vi "safe state action.vi"(8 "error in":errorcluster, 11 "Engine Data Out in":T1={"timed loop timer source"={"Processor"=0, "Priority"=0, "timing source dt"=0, "timer source"=refnum}, "control loop data"={"engine tag bus"={"Double"=[], "Single"=[], "I64"=[], "I32"=[], "I16"=[], "I8"=[], "U64"=[], "U32"=[], "U16"=[], "U8"=[], "Boolean"=[], "String"=[], "Array of Double"=[], "Array of Single"=[], "Array of I64"=[], "Array of I32"=[], "Array of I16"=[], "Array of I8"=[], "Array of U64"=[], "Array of U32"=[], "Array of U16"=[], "Array of U8"=[], "Array of Boolean"=[], "Array of String"=[]}, "engine schedule"={"module run flags"=[], "decimation schedule"={"decimations"=[], "offsets"=[]}}, "module information"=[]}, "status reporting"={"late? index (bool)"=-1, "late count index (U32)"=-1, "dt (ns) index (U64)"=-1}} {"control loop data"."module information"."GUID"."Lo" format="%.0x"; "control loop data"."module information"."GUID"."Hi" format="%.0x"}) -> (0 "error out":errorcluster, 3 "Engine Data Out out":T1={"timed loop timer source"={"Processor"=0, "Priority"=0, "timing source dt"=0, "timer source"=refnum}, "control loop data"={"engine tag bus"={"Double"=[], "Single"=[], "I64"=[], "I32"=[], "I16"=[], "I8"=[], "U64"=[], "U32"=[], "U16"=[], "U8"=[], "Boolean"=[], "String"=[], "Array of Double"=[], "Array of Single"=[], "Array of I64"=[], "Array of I32"=[], "Array of I16"=[], "Array of I8"=[], "Array of U64"=[], "Array of U32"=[], "Array of U16"=[], "Array of U8"=[], "Array of Boolean"=[], "Array of String"=[]}, "engine schedule"={"module run flags"=[], "decimation schedule"={"decimations"=[], "offsets"=[]}}, "module information"=[]}, "status reporting"={"late? index (bool)"=-1, "late count index (U32)"=-1, "dt (ns) index (U64)"=-1}} {"control loop data"."module information"."GUID"."Lo" format="%.0x"; "control loop data"."module information"."GUID"."Hi" format="%.0x"})   [LabVIEW 2013, in "main engine.lvlib"]
uses:
  main engine/main engine.lvlib
  Engine Data.ctl
  <vilib>/NI/Module Timing Source/timing source/TBM timing source.lvclass
  timed loop timing sources.ctl
  control loop data.ctl
  <vilib>/NI/Tag Bus/table/data table.ctl
  engine run schedule.ctl
  engine decimation schedule.ctl
  full module data.ctl
  <vilib>/NI/Tag Bus Module Framework/runtime/TBM module execution interface.lvclass
  module run state.ctl
  async executor/asynchronous executor reference.ctl
  async executor/message to executor.ctl
  async command notification.ctl
  async error info.ctl
  <vilib>/NI/Tag Bus Module Framework/runtime/error classification.ctl
  <vilib>/NI/Tag Bus Module Framework/module configuration/TBM module configuration.lvclass
  <vilib>/NI/Configuration Framework/serializable configuration/Numeric GUID.ctl
  module method data.ctl
  <vilib>/NI/Tag Bus/table/transfer specification.ctl
  <vilib>/NI/Tag Bus/tag/Data Type.ctl
  fault handling spec.ctl
  Configuration/Error Actions.ctl
  status reporting data.ctl
  <vilib>/NI/Tag Bus/table/transfer table data.vi
  <vilib>/NI/Tag Bus/table/data table.lvlib
  <vilib>/NI/Tag Bus/tag/tag descriptor.lvclass
  Configuration/Standard Engine Configuration.lvclass
  async executor/async executor.lvlib
  <vilib>/NI/Configuration Framework/serializable configuration/NISE_CEF_serializable configuration.lvclass
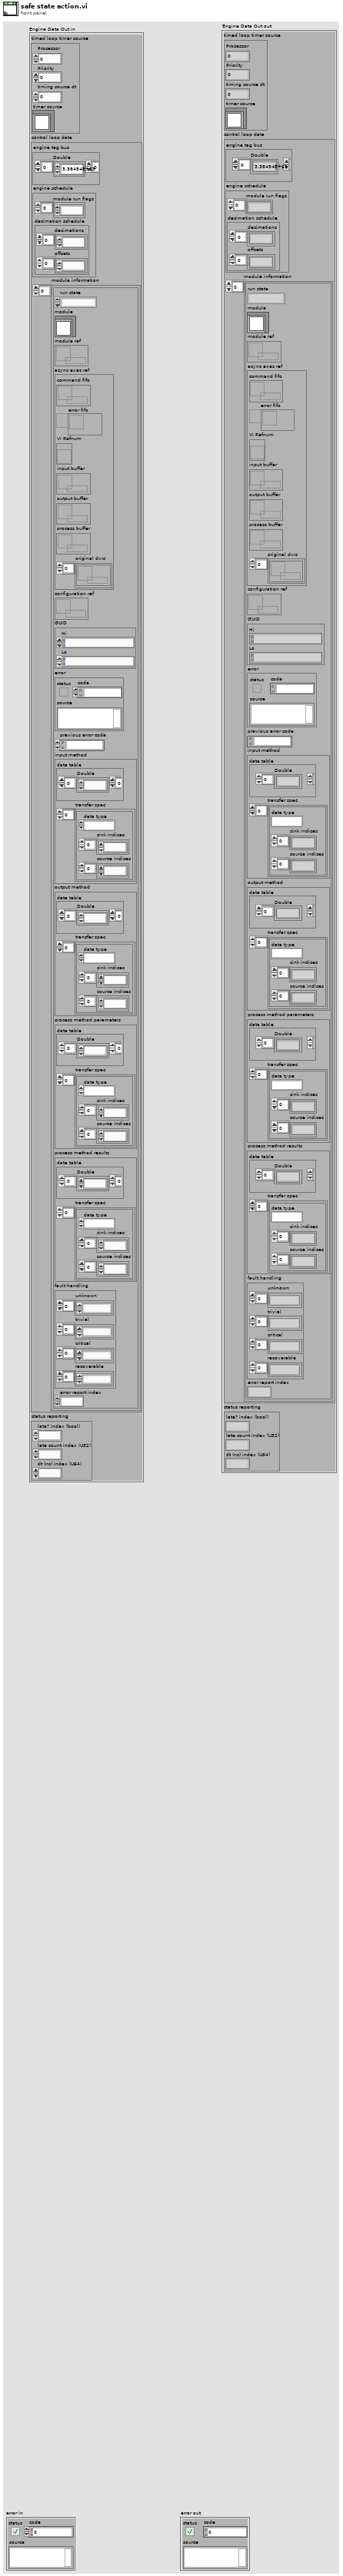
[diagram p1: front panel]
types:
  T1 = typedef "main engine.lvlib/Engine Data.ctl" = cluster{"timed loop timer source":T2, "control loop data":T3, "status reporting":T16}
  T2 = typedef "main engine.lvlib/timed loop timing sources.ctl" = cluster{"Processor":i32, "Priority":i32, "timing source dt":u32, "timer source":refnum<class "TBM timing source.lvclass">}
  T3 = typedef "main engine.lvlib/control loop data.ctl" = cluster{"engine tag bus":T4, "engine schedule":T5, "module information":T7[]}
  T4 = typedef "tag bus.lvlib/data table.lvlib/data table.ctl" = cluster{"Double":dbl[], "Single":sgl[], "I64":i64[], "I32":i32[], "I16":i16[], "I8":i8[], "U64":u64[], "U32":u32[], "U16":u16[], "U8":u8[], "Boolean":bool[], "String":string[], "Array of Double":cluster{"DBL Array":dbl[]}[], "Array of Single":cluster{"SGL Array":sgl[]}[], "Array of I64":cluster{"I64 Array":i64[]}[], "Array of I32":cluster{"I32 Array":i32[]}[], "Array of I16":cluster{"I16 Array":i16[]}[], "Array of I8":cluster{"I8 Array":i8[]}[], "Array of U64":cluster{"U64 Array":u64[]}[], "Array of U32":cluster{"U32 Array":u32[]}[], "Array of U16":cluster{"U16 Array":u16[]}[], "Array of U8":cluster{"U8 Array":u8[]}[], "Array of Boolean":cluster{"Boolean Array":bool[]}[], "Array of String":cluster{"String Array":string[]}[]}
  T5 = typedef "main engine.lvlib/engine run schedule.ctl" = cluster{"module run flags":u8[], "decimation schedule":T6}
  T6 = typedef "main engine.lvlib/engine decimation schedule.ctl" = cluster{"decimations":u16[], "offsets":u16[]}
  T7 = typedef "main engine.lvlib/full module data.ctl" = cluster{"run state":T8, "module":refnum<class "TBM module execution interface.lvclass">, "module ref":refnum<data-value>, "async exec ref":T9, "configuration ref":refnum<data-value>, "GUID":T10, "error":errorcluster, "previous error code":i32, "input method":T11, "output method":T11, "process method parameters":T11, "process method results":T11, "fault handling":T14, "error report index ":i32}
  T8 = typedef "main engine.lvlib/module run state.ctl" = enum16{"sync", "async"}
  T9 = typedef "async executor.lvlib/asynchronous executor reference.ctl" = cluster{"command fifo":refnum<k33>, "error fifo":refnum<k33>, "VI Refnum":refnum<vi>, "input buffer":refnum<k33>, "output buffer":refnum<k33>, "process buffer":refnum<k33>, "original dvrs":refnum<data-value>[]}
  T10 = typedef "NISE_CEF_serializable configuration.lvclass/Numeric GUID.ctl" = cluster{"Hi":u64, "Lo":u64}
  T11 = typedef "main engine.lvlib/module method data.ctl" = cluster{"data table":T4, "transfer spec":T12[]}
  T12 = typedef "tag bus.lvlib/data table.lvlib/transfer specification.ctl" = cluster{"data type":T13, "sink indices":i32[], "source indices":i32[]}
  T13 = typedef "tag bus.lvlib/tag descriptor.lvclass/Data Type.ctl" = enum16{"Double", "Single", "I64", "I32", "I16", "I8", "U64", "U32", "U16", "U8", "Boolean", "String", "Array of Double", "Array of Single", "Array of I64", "Array of I32", "Array of I16", "Array of I8", "Array of U64", "Array of U32", "Array of U16", "Array of U8", "Array of Boolean", "Array of String"}
  T14 = typedef "main engine.lvlib/fault handling spec.ctl" = cluster{"unknown":T15[], "trivial":T15[], "critical":T15[], "recoverable":T15[]}
  T15 = typedef "Standard Engine Configuration.lvclass/Error Actions.ctl" = enum16{"Clear", "Notify", "Stop Component", "Stop Engine", "Safe State", "Attempt Recovery"}
  T16 = typedef "main engine.lvlib/status reporting data.ctl" = cluster{"late? index (bool)":i32, "late count index (U32)":i32, "dt (ns) index (U64)":i32}
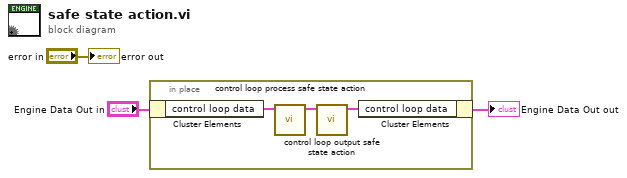
[diagram p0: block diagram]
diagram:
  n1 = in-place {
    n2 = in-place-cluster #1("Engine Data Out in") -> ("control loop data"=w5:T3)
    n3 = call "control loop process safe state action.vi"("control loop data in"=w5) -> ("control loop data out"=w4:T3)  [unwired: 10 in]
    n4 = call "control loop output safe state action.vi"("control loop data in"=w4) -> ("control loop data out"=w6:T3)  [unwired: 10 in]
    n5 = in-place-cluster #1("control loop data"=w6) -> (→"Engine Data Out out":T1)
  }
  "error out" <- "error in"
